vi "Observer Count.vi"(11 "Observer Pattern Actor Interface.lvlib:Subject.lvclass":refnum<class "Subject.lvclass">) -> (1 "size(s)":i32, 3 "Subject out":refnum<class "Subject.lvclass">)   [LabVIEW 2013, in "Observer Pattern Actor Interface.lvlib" / "Subject.lvclass"]
uses:
  Subject.lvclass
  Subject.lvclass/Subject.ctl
  Global 2.vi
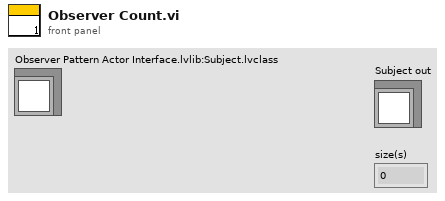
[diagram p1: front panel]
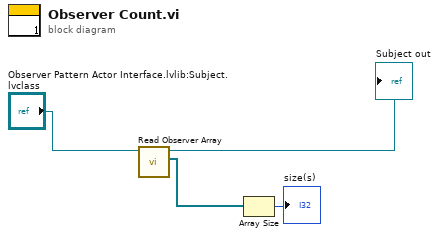
[diagram p0: block diagram]
diagram:
  n1 = call "Read Observer Array.vi"("Subject in"="Observer Pattern Actor Interface.lvlib:Subject.lvclass") -> ("Observer Array"=w2:refnum<class "Message Enqueuer.lvclass">[], "Subject out"=→"Subject out":refnum<class "Subject.lvclass">)  [unwired: 8 in, 1 out]
  n2 = Array Size(array=w2) -> (size(s)=→"size(s)":i32)
